vi "Read Roles.vi"(8 "error in (no error)":errorcluster, 11 "PrepareRollToPassPlay in":refnum<class "PrepareRollToPassPlay.lvclass">) -> (0 "error out":errorcluster, 2 "Roles":T1, 3 "PrepareRollToPassPlay out":refnum<class "PrepareRollToPassPlay.lvclass">)   [LabVIEW 2023, in "PrepareRollToPassPlay.lvclass"]
uses:
  PrepareRollToPassPlay.lvclass
  PreparePassReceiverRole_class/PreparePassReceiverRole.lvclass
  PrepareRollToPassReceiverRole_class/PrepareRollToPassReceiverRole.lvclass
  PrepareRollToPassRollerRole_class/PrepareRollToPassRollerRole.lvclass
  PrepareRollToPassPlay.lvclass/PrepareRollToPassPlay.ctl
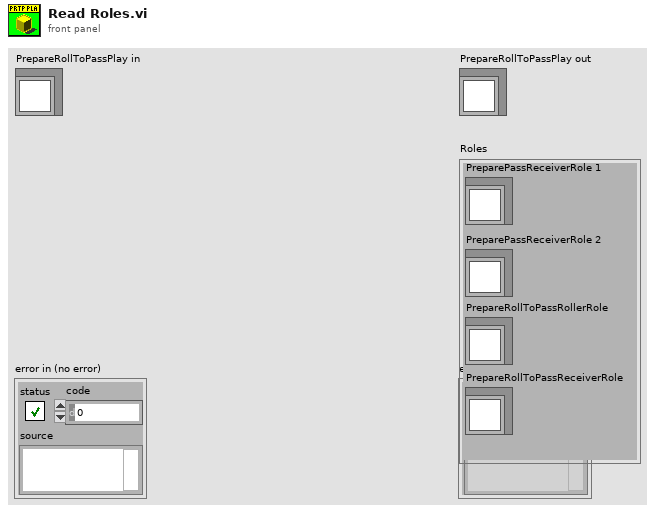
[diagram p1: front panel]
types:
  T1 = cluster{"PreparePassReceiverRole 1":refnum<class "PreparePassReceiverRole.lvclass">, "PreparePassReceiverRole 2":refnum<class "PreparePassReceiverRole.lvclass">, "PrepareRollToPassReceiverRole":refnum<class "PrepareRollToPassReceiverRole.lvclass">, "PrepareRollToPassRollerRole":refnum<class "PrepareRollToPassRollerRole.lvclass">}
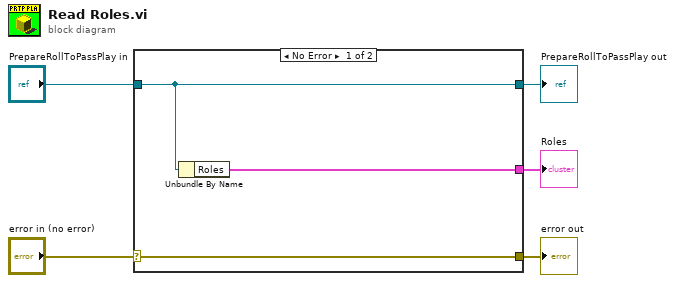
[diagram p0: block diagram]
diagram:
  n1 = case shown="No Error" "error in (no error)" {
    selector: "error in (no error)" -> [w8 w9]
    tunnel: [w8 w9] -> w4
    tunnel: [w7 w10] -> w2
    tunnel: "PrepareRollToPassPlay in" -> [w7 w10]
    tunnel: [w6 _] -> w1
    frame No Error {
      n2 = Unbundle By Name(w7) -> ("Roles"=w6:T1)
    }
    frame Error {
    }
  }
  "error out" <- w4
  "PrepareRollToPassPlay out" <- w2
  "Roles" <- w1
